vi "Retrieve Inline Section configuration properties (objects).vi"(8 "error in":errorcluster, 11 "section item ref in":T2 format="%.0x") -> (0 "error out":errorcluster, 1 "status channel configuration":map{string, map{string, i32}}(c390), 2 "configuration properties":T3[](array[typedef]), 3 "section item ref out":T2 format="%.0x", 4 "Found":bool, 5 "inline vs group data refs":T1 {"item refs - info" format="%.0x"; "item refs - data" format="%.0x"})   [LabVIEW 2019, in "HLA Custom Device System Explorer.lvlib"]
uses:
  HLA Custom Device System Explorer.lvlib
  <vilib>/NI VeriStand/Custom Device API/Custom Device Item Ref.ctl
  Shared/object_attribute_configuration.ctl
  Shared/inline_vs_group_refs.ctl
  Shared/Constants.vi
  <vilib>/NI VeriStand/Custom Device API/Get Item Property (String).vi
  <vilib>/NI VeriStand/Custom Device API/Custom Device API.lvlib
  Shared/HLA Custom Device Shared.lvlib
  <vilib>/NI VeriStand/Custom Device Tools/Custom Device Utility Library/Custom Device Utility Library.lvlib
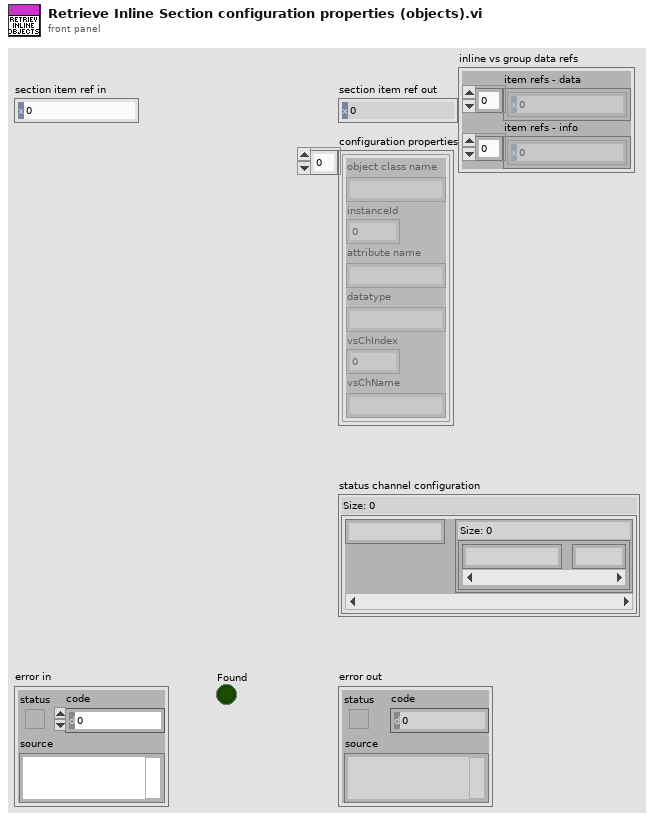
[diagram p1: front panel]
types:
  T1 = typedef "HLA Custom Device Shared.lvlib/inline_vs_group_refs.ctl" = cluster{"item refs - data":T2[], "item refs - info":T2[]}
  T2 = typedef "Custom Device API.lvlib/Custom Device Item Ref.ctl" = u64
  T3 = typedef "HLA Custom Device Shared.lvlib/object_attribute_configuration.ctl" = cluster{"object class name":string, "instanceId":i32, "attribute name":string, "datatype":string, "vsChIndex":i32, "vsChName":string}
  T4 = typedef "Custom Device API.lvlib/Custom Device Item Info.ctl" = cluster{"Name":string, "Is Channel":bool, "GUID":string, "Is Waveform":bool}
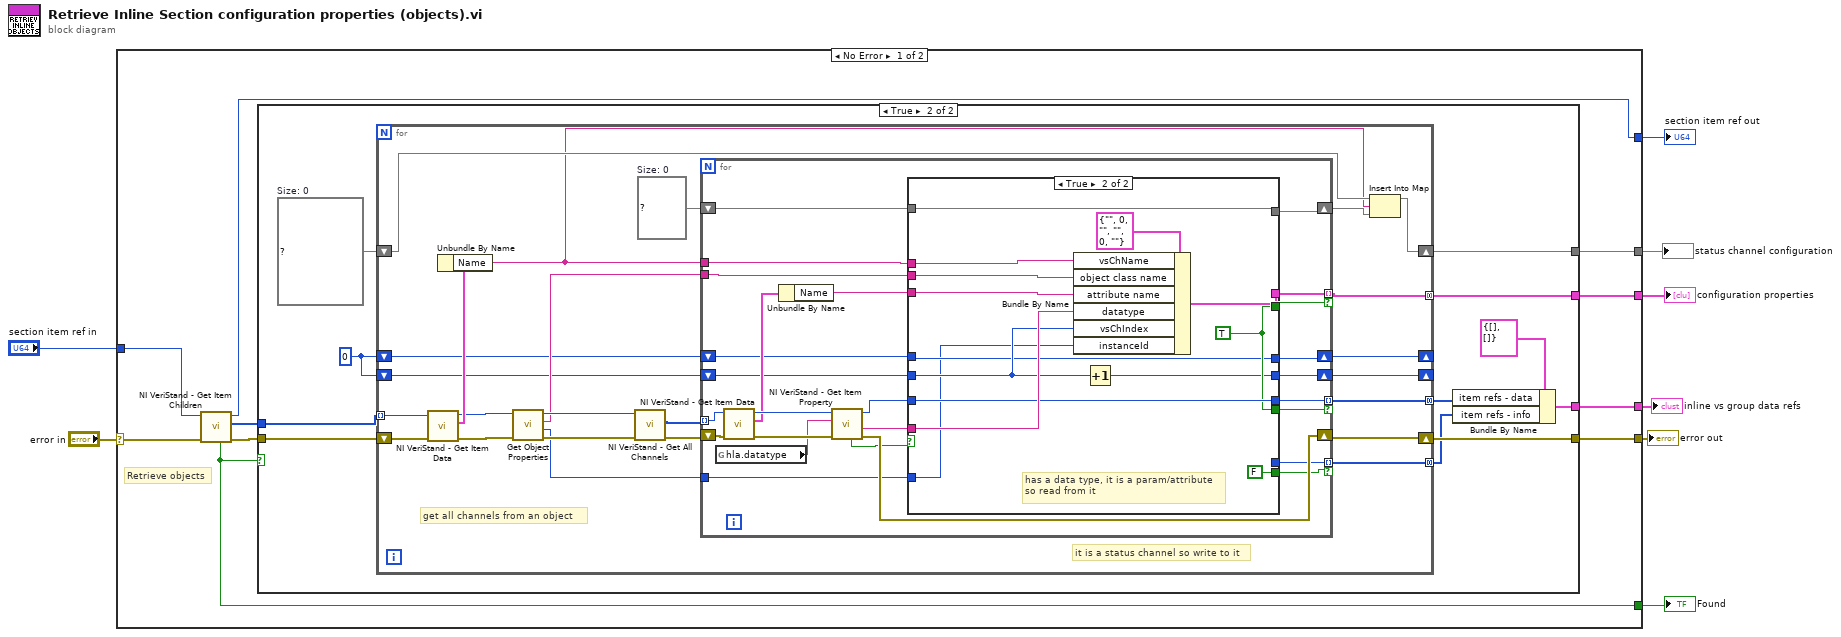
[diagram p0: block diagram]
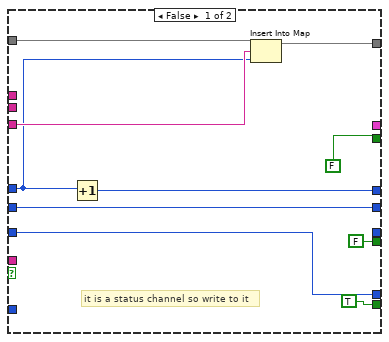
[diagram p3: hidden frame]
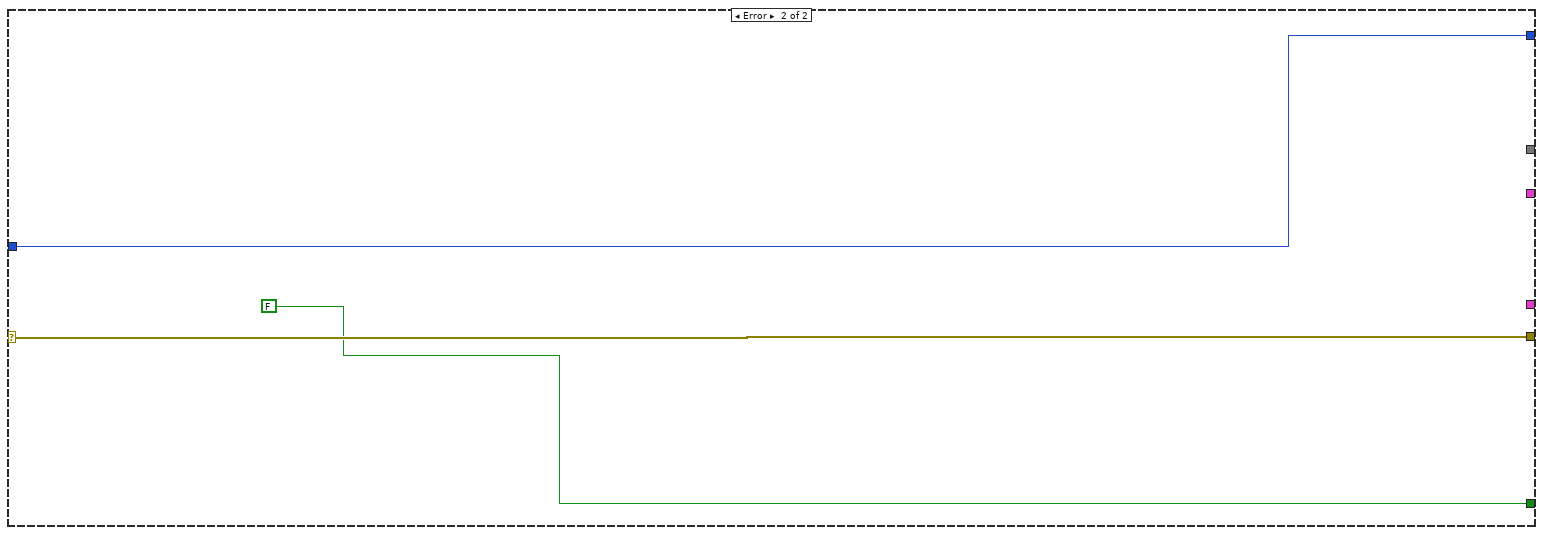
[diagram p4: hidden frame]
diagram:
  n1 = case shown="No Error" "error in" {
    selector: "error in" -> [w15 w106]
    tunnel: [w10 w106] -> w7
    tunnel: [w14 w107] -> w6
    tunnel: "section item ref in" -> [w16 w107]
    tunnel: [w11 FALSE ("Found")] -> w4
    tunnel: [w13 _] -> w3
    tunnel: [w12 _] -> w2
    tunnel: [w9 _] -> w1
    frame No Error {
      # "Retrieve objects"
      n2 = call <vilib>:"NI VeriStand - Get Item Children.vi"("error in (no error)"=w15, "Item Ref in"=w16) -> ("error out"=w17:errorcluster, "Child Refs"=w18:T2[], "Item Ref out"=w14:T2, "Found"=w11:bool)  [unwired: 6 in]
      n3 = case shown="True" w11 {
        tunnel: w18 -> [_ w30]
        tunnel: w17 -> [w19 w29]
        tunnel: [_ w28] -> w13
        tunnel: [_ w26] -> w12
        tunnel: [w19 w24] -> w10
        tunnel: [_ w20] -> w9
        frame False {
        }
        frame True {
          w25 = 0
          w27 = map{string, map{string, i32}} {}  # Size: 0
          n4 = for {
            shift-right: [w46] -> w24
            shift-left: w29 -> [w53]
            tunnel: w30 -> [w52] mode=indexing
            tunnel: [w47] -> w28 mode=concatenating
            shift-right: [w48] -> w26
            shift-left: w27 -> [w50]
            tunnel: [w37] -> w22 mode=concatenating
            tunnel: [w36] -> w21 mode=concatenating
            shift-right: [w33] -> _
            shift-left: w25 -> [w35]
            shift-right: [w32] -> _
            shift-left: w25 -> [w34]
            w51 = map{string, i32} {}  # Size: 0
            # "it is a status channel so write to it"
            # "get all channels from an object"
            n5 = call <vilib>:"NI VeriStand - Get Item Data.vi"("error in (no error)"=w53, "Item Ref in"=w52) -> ("error out"=w43:errorcluster, "Item Info"=w54:T4, "Item Ref out"=w42:T2)  [unwired: 6 in, 1 out]
            n6 = Unbundle By Name(w54) -> ("Name"=w38:string)
            n7 = call "Get Object Properties.vi"("error in (no error)"=w43, "Item Ref in"=w42) -> ("error out"=w40:errorcluster, "instance id"=w31:i32, "class name"=w39:string, "Item Ref out"=w41:T2)  [unwired: 6 in]
            n8 = call <vilib>:"NI VeriStand - Get All Channels.vi"("error in"=w40, "Section Ref in"=w41) -> ("error out"=w44:errorcluster, "Channel Refs"=w45:T2[])  [unwired: 6 in, 2 out]
            n9 = for {
              tunnel: w39 -> [w75]
              tunnel: w45 -> [w80] mode=indexing
              tunnel: [w74] -> w47 mode=indexing if=w66
              shift-right: [w73] -> w46
              shift-left: w44 -> [w79]
              shift-right: [w67] -> w49
              shift-left: w51 -> [w68]
              tunnel: w38 -> [w65]
              tunnel: [w63] -> w37 mode=indexing if=w62
              tunnel: [w61] -> w36 mode=indexing if=w60
              shift-right: [w57] -> w33
              shift-left: w35 -> [w59]
              shift-right: [w56] -> w32
              shift-left: w34 -> [w58]
              tunnel: w31 -> [w55]
              n10 = global read "Constants.vi" "hla.datatype"() -> (w76:string)
              n11 = call <vilib>:"NI VeriStand - Get Item Data.vi"("error in (no error)"=w79, "Item Ref in"=w80) -> ("error out"=w77:errorcluster, "Item Info"=w71:T4, "Item Ref out"=w78:T2)  [unwired: 6 in, 1 out]
              n12 = Unbundle By Name(w71) -> ("Name"=w70:string)
              n13 = call-poly <vilib>:"NI VeriStand - Get Item Property.vi"("error in (no error)"=w77, "Property Name"=w76, "Item Ref in"=w78) -> ("error out"=w73:errorcluster, "Value"=w72:string, "Item Ref out"=w64:T2, "Found?"=w69:bool)  [unwired: 5 in]
              n14 = case shown="True" w69 {
                tunnel: w75 -> [_ w104]
                tunnel: [_ w103] -> w74
                tunnel: w72 -> [_ w102]
                tunnel: w70 -> [w89 w101]
                tunnel: w68 -> [w90 w100]
                tunnel: [w88 w100] -> w67
                tunnel: [FALSE w96] -> w66
                tunnel: w65 -> [_ w98]
                tunnel: w64 -> [w86 w97]
                tunnel: [_ w97] -> w63
                tunnel: [FALSE w96] -> w62
                tunnel: [w86 _] -> w61
                tunnel: [TRUE FALSE] -> w60
                tunnel: w59 -> [w83 w92]
                tunnel: w58 -> [w81 w94]
                tunnel: [w82 w92] -> w57
                tunnel: [w81 w93] -> w56
                tunnel: w55 -> [_ w91]
                frame False {
                  # "it is a status channel so write to it"
                  n15 = Increment(x=w83) -> (x+1=w82:i32)
                  n16 = Insert Into Map(map in=w90, key=w89, value=w83) -> (map out=w88:map{string, i32})  [unwired: 2 out]
                }
                frame True {
                  w96 = TRUE
                  # "has a data type, it is a param/attribute\nso read from it"
                  n17 = Bundle By Name(cluster=T3 {"object class name"="", "instanceId"=0, "attribute name"="", "datatype"="", "vsChIndex"=0, "vsChName"=""}, "vsChName"=w98, "object class name"=w104, "attribute name"=w101, "datatype"=w102, "vsChIndex"=w94, "instanceId"=w91) -> (w103:T3)
                  n18 = Increment(x=w94) -> (x+1=w93:i32)
                }
              }
            }
            n19 = Insert Into Map(map in=w50, key=w38, value=w49) -> (map out=w48:map{string, map{string, i32}})  [unwired: 2 out]
          }
          n20 = Bundle By Name(cluster=T1 {"item refs - data"=[], "item refs - info"=[]} ("inline vs group data refs"), "item refs - data"=w22, "item refs - info"=w21) -> (w20:T1)
        }
      }
    }
    frame Error {
    }
  }
  "error out" <- w7
  "section item ref out" <- w6
  "Found" <- w4
  "configuration properties" <- w3
  "status channel configuration" <- w2
  "inline vs group data refs" <- w1
